vi "Update Summation.vi"(7 "Data Set":dbl[](array[numeric]), 8 "tolerance":dbl=0.0001, 9 "x0":dbl, 10 "x":dbl, 11 "summation in":dbl) -> (3 "summation out":dbl)   [LabVIEW 2020, in "NI_PtbyPt.lvlib"]
uses:
  NI_PtbyPt.lvlib
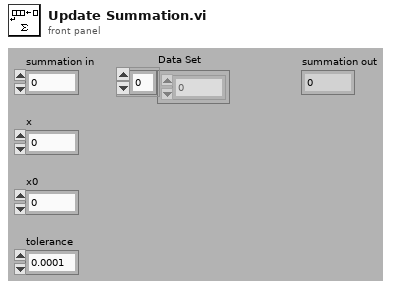
[diagram p1: front panel]
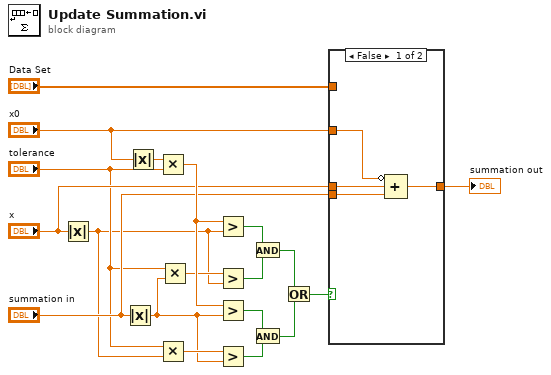
[diagram p0: block diagram]
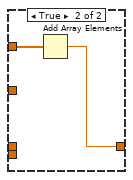
[diagram p2: hidden frame]
diagram:
  n1 = Absolute Value(x="x") -> (abs(x)=w1:dbl)
  n2 = Absolute Value(x="summation in") -> (abs(x)=w4:dbl)
  n3 = Absolute Value(x="x0") -> (abs(x)=w5:dbl)
  n4 = Multiply(x=w5, y="tolerance") -> (x*y=w17:dbl)
  n5 = Multiply(x="tolerance", y=w1) -> (x*y=w15:dbl)
  n6 = Multiply(x="tolerance", y=w4) -> (x*y=w16:dbl)
  n7 = Greater?(x=w17, y=w1) -> (0:w19:bool)
  n8 = Greater?(x=w16, y=w1) -> (0:w18:bool)
  n9 = Greater?(x=w17, y=w4) -> (0:w14:bool)
  n10 = Greater?(x=w15, y=w4) -> (0:w13:bool)
  n11 = And(x=w19, y=w18) -> (x .and. y?=w12:bool)
  n12 = And(x=w14, y=w13) -> (x .and. y?=w11:bool)
  n13 = Or(x=w12, y=w11) -> (x .or. y?=w10:bool)
  n14 = case shown="False" w10 {
    tunnel: "Data Set" -> [_ w25]
    tunnel: [w20 w24] -> w6
    tunnel: "x0" -> [w23 _]
    tunnel: "summation in" -> [w21 _]
    tunnel: "x" -> [w22 _]
    frame False {
      n15 = Compound Arithmetic op=ADD(invert w23, w22, w21) -> (w20:dbl)
    }
    frame True {
      n16 = Add Array Elements(numeric array=w25) -> (sum=w24:dbl)
    }
  }
  "summation out" <- w6
